vi "LVAPT-GIT-Push.vi"(11 "path":path) -> ()   [LabVIEW 2019]
uses:
  <vilib>/Hampel Software Engineering/Git API/Git API/GIT-api.lvclass/GIT-api.ctl
  <vilib>/Hampel Software Engineering/Git API/Git API/Accessors/GIT-Set Working Dir.vi
  <vilib>/Hampel Software Engineering/Git API/Git API/GIT-api.lvclass
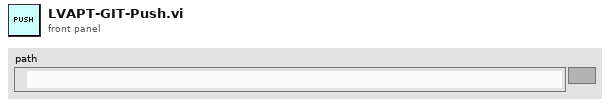
[diagram p1: front panel]
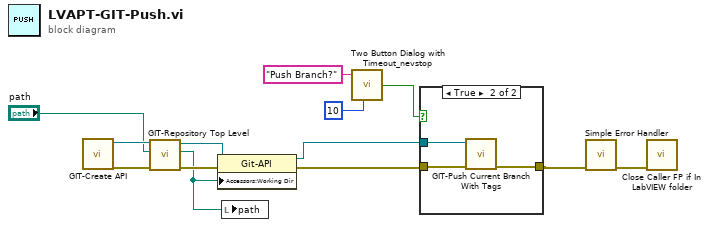
[diagram p0: block diagram]
diagram:
  n1 = call <vilib>:"GIT-Create API.vi"() -> ("error out"=w10:errorcluster, "git-api out"=w11:refnum<class "GIT-api.lvclass">)  [unwired: 10 in]
  n2 = call <vilib>:"GIT-Repository Top Level.vi"("error in"=w10, "Current Path"="path", "git-api in"=w11) -> ("error out"=w13:errorcluster, "Repo Top Level Path"=w1:path, "git-api out"=w12:refnum<class "GIT-api.lvclass">)  [unwired: 6 in]
  n3 = property class="Git-API"(reference=w12, error in=w13, "Accessors:Working Dir"=w1) -> (reference out=w8:refnum<class "GIT-api.lvclass">, error out=w9:errorcluster)
  n4 = local write "path"(w1) -> ()
  n5 = call <userlib>:"Two Button Dialog with Timeout_nevstop.vi"("message"="Push Branch?", "F Timeout(-1 s)"=10) -> ("T button?"=w4:bool)  [unwired: 3 in]
  n6 = case shown="True" w4 {
    tunnel: w9 -> [w14 w17]
    tunnel: [w14 w16] -> w2
    tunnel: w8 -> [_ w15]
    frame False {
    }
    frame True {
      n7 = call <vilib>:"GIT-Push Current Branch With Tags.vi"("error in"=w17, "Git-API in"=w15) -> ("error out"=w16:errorcluster)  [unwired: 8 in, 1 out]
    }
  }
  n8 = call <vilib>:"Simple Error Handler.vi"("error in (no error)"=w2) -> ("error out"=w3:errorcluster)  [unwired: 4 in, 4 out]
  n9 = call "Close Caller FP if In LabVIEW folder.vi"("error in (no error)"=w3) -> ()  [unwired: 10 in, 1 out]
